vi "Stop Loop.vi"(8 "error in (no error)":errorcluster, 11 "FHPP in":refnum<class "FHPP.lvclass">) -> (0 "error out":errorcluster)   [LabVIEW 2022 SP3, in "FHPP.lvclass"]
uses:
  FHPP.lvclass
  FHPP.lvclass/FHPP.ctl
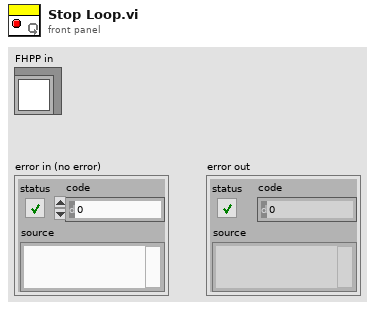
[diagram p1: front panel]
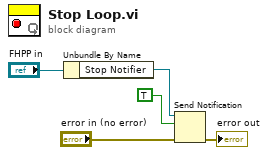
[diagram p0: block diagram]
diagram:
  n1 = Unbundle By Name("FHPP in") -> ("Stop Notifier"=w2:refnum<notifier>)
  n2 = Send Notification(notification=TRUE, notifier=w2, error in (no error)="error in (no error)") -> (error out=→"error out":errorcluster)  [unwired: 1 out]
